vi "Close.vi"(8 "error in":errorcluster, 11 "Instrument Handle In":i32) -> (0 "error out":errorcluster)   [LabVIEW 2020, in "ZTScopeM.lvlib"]
doc: "Close the passed in communication session. This does not affect other communication sessions that may have been opened."
uses:
  ZTScopeM.lvlib
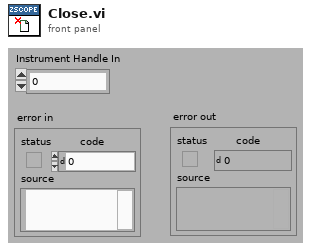
[diagram p1: front panel]
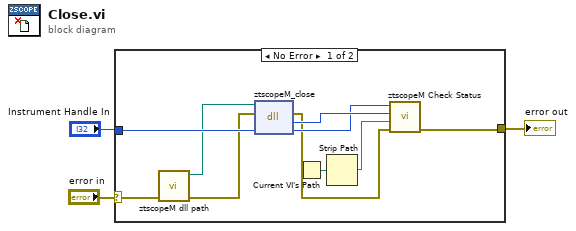
[diagram p0: block diagram]
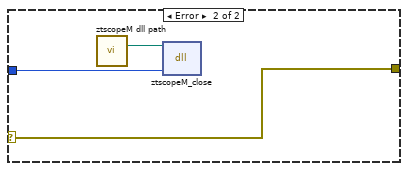
[diagram p2: hidden frame]
diagram:
  n1 = case shown="No Error" "error in" {
    selector: "error in" -> [w7 w16]
    tunnel: [w8 w16] -> w1
    tunnel: "Instrument Handle In" -> [w13 w15]
    frame No Error {
      n2 = call "ztscopeM dll path.vi"("error in (no error)"=w7) -> ("error out"=w5:errorcluster, "<instrument>.dll path"=w6:path)  [unwired: 9 in]
      n3 = dll-call lib="C:/Program Files (x86)/National Instruments/LabVIEW 2013/instr.lib/ztscopem/ztscopeM.dll" fn="ztscopeM_close"(path in=w6, error in=w5, "instrumentHandle"=w13) -> (error out=w4:errorcluster, "return type"=w10:i32, "instrumentHandle"=w9:i32)  [unwired: 1 in, 1 out]
      n4 = Current VI's Path() -> (path=w12:path)
      n5 = Strip Path(path=w12) -> (name=w11:string)  [unwired: 1 out]
      n6 = call "ztscopeM Check Status.vi"("error in"=w4, "name of VI"=w11, "status (return code)"=w10, "instrument handle in"=w9) -> ("error out"=w8:errorcluster)  [unwired: 2 in, 1 out]
    }
    frame Error {
      n7 = call "ztscopeM dll path.vi"() -> ("<instrument>.dll path"=w14:path)  [unwired: 10 in, 1 out]
      n8 = dll-call lib="C:/Program Files (x86)/National Instruments/LabVIEW 2013/instr.lib/ztscopem/ztscopeM.dll" fn="ztscopeM_close"(path in=w14, "instrumentHandle"=w15) -> ()  [unwired: 4 in, 2 out]
    }
  }
  "error out" <- w1
